vi "niRFSysCalReader Interpolator.vi"(4 "Power (dBm)":dbl, 6 "Frequency (Hz)":dbl, 8 "error in":errorcluster, 11 "niRFSysCalReader Handle":T1) -> (0 "error out":errorcluster, 2 "Interpolated Pathloss (dB)":dbl, 3 "niRFSysCalReader Handle out":T1)   [LabVIEW 2016, in "niRFSysCalReader.lvlib"]
doc: "Performs an interpolation on the Calibration Data."
uses:
  niRFSysCalReader.lvlib
  _INCLUDES/niRFSysCalReader Handle.ctl
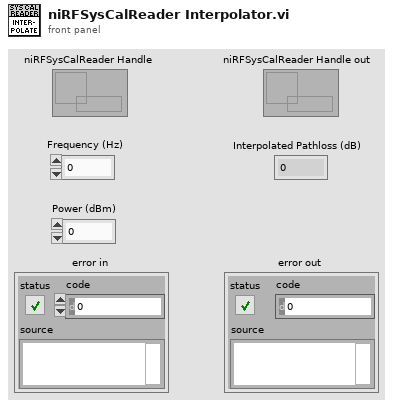
[diagram p1: front panel]
types:
  T1 = typedef "niRFSysCalReader.lvlib/niRFSysCalReader Handle.ctl" = refnum<data-value>
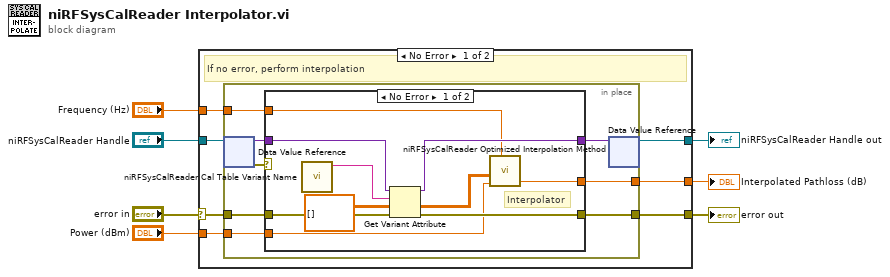
[diagram p0: block diagram]
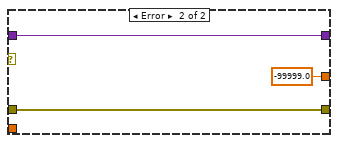
[diagram p2: hidden frame]
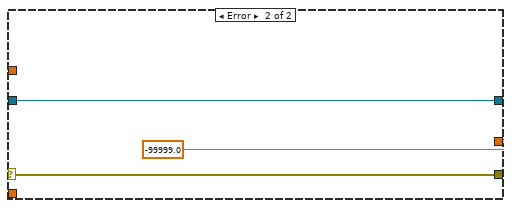
[diagram p3: hidden frame]
diagram:
  n1 = case shown="No Error" "error in" {
    selector: "error in" -> [w13 w36]
    tunnel: "Frequency (Hz)" -> [w8 _]
    tunnel: "Power (dBm)" -> [w9 _]
    tunnel: [w10 -99999.0] -> w5
    tunnel: [w12 w36] -> w4
    tunnel: "niRFSysCalReader Handle" -> [w14 w38]
    tunnel: [w11 w38] -> w2
    frame No Error {
      # "If no error, perform interpolation"
      n2 = in-place {
        in-place-border: w13 -> [w21]
        in-place-border: [w19] -> w12
        in-place-border: [w18] -> w10
        in-place-border: w9 -> [w17]
        in-place-border: w8 -> [w16]
        n3 = in-place-dvr #1(w14) -> (w22:variant, w15:errorcluster)
        n4 = case shown="No Error" w15 {
          tunnel: w22 -> [w32 w35]
          tunnel: w21 -> [w30 w34]
          tunnel: [w29 w35] -> w20
          tunnel: [w28 w34] -> w19
          tunnel: [w27 -99999.0 ("External Attenuation, dB")] -> w18
          tunnel: w17 -> [w25 _]
          tunnel: w16 -> [w24 _]
          frame No Error {
            # "Interpolator"
            n5 = call "niRFSysCalReader Cal Table Variant Name.vi"() -> ("Calibration Table Name"=w23:string)  [unwired: 11 in]
            n6 = Get Variant Attribute(Variant=w32, name=w23, default value (empty Variant)=dbl[][] [], error in=w30) -> (duplicate Variant=w29:variant, value=w26:dbl[][], error out=w28:errorcluster)  [unwired: 1 out]
            n7 = call "niRFSysCalReader Optimized Interpolation Method.vi"("Table (frequency, power, pathloss)"=w26, "Max Input Power, dBm"=w25, "Center Frequency, Hz"=w24) -> ("External Attenuation, dB"=w27:dbl)  [unwired: 2 in, 2 out]
          }
          frame Error {
          }
        }
        n8 = in-place-dvr #1(w20) -> (w11:T1)  [unwired: 1 out]
      }
    }
    frame Error {
    }
  }
  "error out" <- w4
  "Interpolated Pathloss (dB)" <- w5
  "niRFSysCalReader Handle out" <- w2
